vi "Obtain frame size in bytes.vi"(8 "error in (no error)":errorcluster, 11 "Binary file to read":path=path "C:/Temp/BodyCam.bin") -> (0 "error out":errorcluster, 3 "Frame size (bytes)":i64)   [LabVIEW 2017]
uses:
  Typedefs/Binary Cam data type definition.ctl
  <vilib>/vision/Image Controls.llb/IMAQ Image.ctl
panel:
  out "Rel times when allowed to run to the end (used for validation)":i64[](array[numeric])
  out "Bytes":i32
  out "Locations when allowed to run to the end (used for validation)":i64[](array[numeric])
  out "Image":T1(plugin-control)
  in  "stop":bool
  out "Frame number":i32
  out "Rel time (ms)":u32
  out "Time taken (ms)":u32
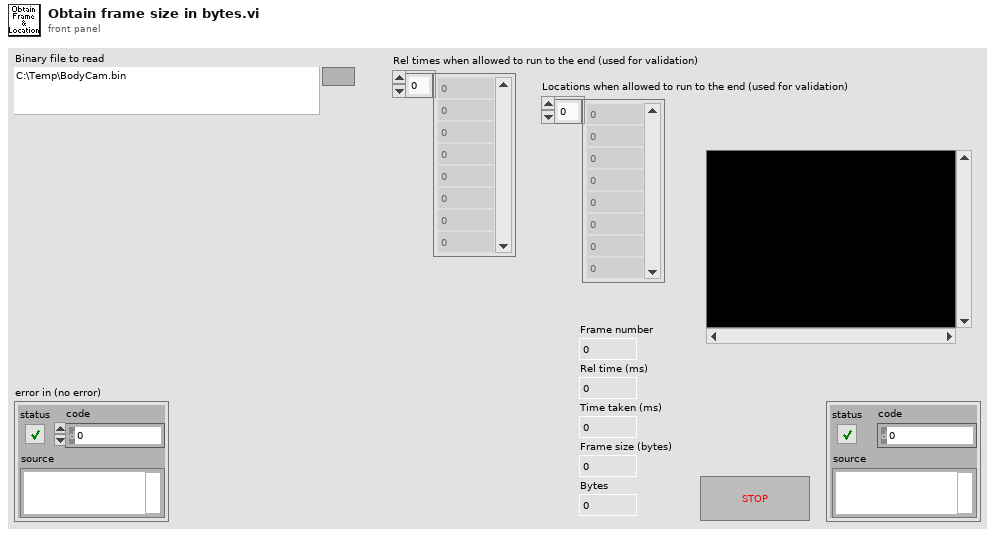
[diagram p1: front panel]
types:
  T1 = typedef "IMAQ Image.ctl" = refnum<image>
  T2 = enum16{"open", "replace", "create", "open or create", "replace or create", "replace or create with confirmation"}
  T3 = typedef "Binary Cam data type definition.ctl" = cluster{"Image":T1, "Rel time":u32}
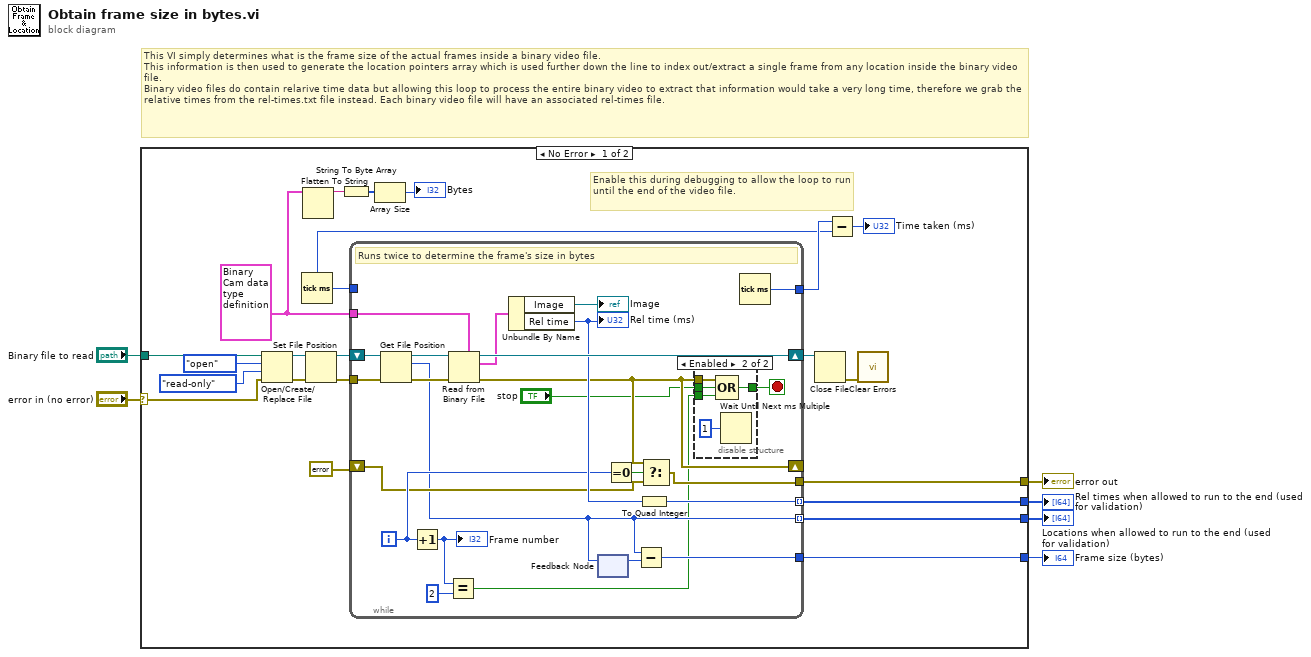
[diagram p0: block diagram]
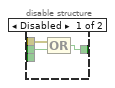
[diagram p2: hidden frame]
diagram:
  # "This VI simply determines what is the frame size of the actual frames inside a binary video file.\nThis information is then used to generate the location pointers array which is used further down the line to index out/extract a single frame from any location inside the binary video file.\nBinary video files do contain relarive time data but allowing this loop to process the entire binary video to extract that information would take a very long time, therefore we grab the relative times from the rel-times.txt file instead. Each binary video file will have an associated rel-times file."
  n1 = case shown="No Error" "error in (no error)" {
    selector: "error in (no error)" -> [w11 w61]
    tunnel: "Binary file to read" -> [w18 _]
    tunnel: [w10 w61] -> w4
    tunnel: [w9 _] -> w3
    tunnel: [w8 _] -> w2
    tunnel: [w7 _] -> w1
    frame No Error {
      w12 = T3 {"Image"=refnum, "Rel time"=0} ("output cluster")
      # "Enable this during debugging to allow the loop to run until the end of the video file."
      n2 = Open/Create/Replace File(file path (use dialog)=w18, error in=w11, operation (0:open)=T2."open", access (0:read/write)=enum16{"read/write", "read-only", "write-only"}."read-only") -> (refnum out=w17:refnum<file>, error out=w16:errorcluster)  [unwired: 2 in, 1 out]
      n3 = Tick Count (ms)() -> (millisecond timer value=w24:u32)
      n4 = Flatten To String(anything=w12) -> (data string=w14:string)  [unwired: 3 in, 2 out]
      n5 = Set File Position(refnum=w17, error in=w16) -> (refnum out=w22:refnum<file>, error out=w21:errorcluster)  [unwired: 2 in]
      n6 = String To Byte Array(string=w14) -> (unsigned byte array=w15:u8[])
      n7 = while {
        tunnel: w21 -> [w46]
        shift-right: [w52] -> w26
        shift-left: w22 -> [w49]
        tunnel: w12 -> [w51]
        tunnel: w24 -> [_]
        tunnel: [w44] -> w25
        tunnel: [w43] -> w9 mode=indexing
        tunnel: [w36] -> w8 mode=indexing
        tunnel: [w40] -> w10
        shift-right: [w41] -> _
        shift-left: errorcluster {"status"=FALSE, "code"=0, "source"=""} ("error out") -> [w38]
        tunnel: [w34] -> w7
        i -> [w39]
        stop <- w50 stop-if-true
        # "Runs twice to determine the frame's size in bytes"
        n8 = Get File Position(4:w46, 7:w49) -> (0:w45:errorcluster, 2:w36:i64, 3:w48:refnum<file>)
        n9 = Increment(x=w39) -> (x+1=w33:i32)
        "Frame number" <- w33
        n10 = Equal?(x=w33, y=2) -> (x = y?=w31:bool)
        n11 = Read from Binary File(5:w51, 8:w45, 11:w48) -> (0:w41:errorcluster, 2:w30:T3, 3:w52:refnum<file>)  [unwired: 3 in, 1 out]
        n12 = Unbundle By Name(w30) -> ("Image"=→"Image":T1, "Rel time"=w47:u32)
        "Rel time (ms)" <- w47
        n13 = feedback-in #1(w36) -> ()
        n14 = feedback #1() -> (w35:i64)  [unwired: 1 in]
        n15 = Equal To 0?(x=w39) -> (x = 0?=w42:bool)
        n16 = Subtract(x=w36, y=w35) -> (x-y=w34:i64)
        n17 = To Quad Integer(1:w47) -> (0:w43:i64)
        n18 = Select(t=w41, s=w42, f=w38) -> (s? t:f=w40:errorcluster)
        n19 = disable-structure shown="Enabled" {
          disable-tunnel: [w55 w60] -> w50
          disable-tunnel: "stop" -> [w54 w59]
          disable-tunnel: w41 -> [w53 w58]
          disable-tunnel: w31 -> [_ w57]
          frame Disabled {
            n20 = Compound Arithmetic op=OR(w53, w54) -> (w55:bool)
          }
          frame Enabled {
            n21 = Compound Arithmetic op=OR(w58, w59, w57) -> (w60:bool)
            n22 = Wait Until Next ms Multiple(millisecond multiple=u32 1) -> ()  [unwired: 1 out]
          }
        }
        n23 = Tick Count (ms)() -> (millisecond timer value=w44:u32)
      }
      n24 = Array Size(array=w15) -> (size(s)=→"Bytes":i32)
      n25 = Close File(refnum=w26) -> (error out=w19:errorcluster)  [unwired: 1 in, 1 out]
      n26 = Subtract(x=w25, y=w24) -> (x-y=→"Time taken (ms)":u32)
      n27 = call <vilib>:"Clear Errors.vi"("error in (no error)"=w19) -> ()  [unwired: 5 in, 2 out]
    }
    frame Error {
    }
  }
  "error out" <- w4
  "Locations when allowed to run to the end (used for validation)" <- w2
  "Frame size (bytes)" <- w1
  "Rel times when allowed to run to the end (used for validation)" <- w3
